vi "TemperatureTest.vi"() -> ()   [LabVIEW 2019]
uses:
  <vilib>/DAQmx/read.llb/DAQmx Read (Analog 1D DBL NChan 1Samp).vi
  <vilib>/DAQmx/create/channels.llb/DAQmx Create Channel (AI-Temperature-RTD).vi
  <vilib>/DAQmx/miscellaneous.llb/DAQmx Fill In Error Info.vi
panel:
  in  "rtd type":i32(ring)=10071 items=["Pt3750"=12481, "Pt3851"=10071, "Pt3911"=12482, "Pt3916"=10069, "Pt3920"=10053, "Pt3928"=12483, "Custom"=10137]
  in  "current excitation value":dbl=0.0009 format="%0.5f"
  in  "r0":dbl=100.0 format="%0.2f"
  in  "current excitation source":i32(ring)=10200 items=["Internal"=10200, "External"=10167, "None"=10230]
  in  "units":i32(ring)=10143 items=["Deg C"=10143, "Deg F"=10144, "Kelvins"=10325, "Deg R"=10145, "From Custom Scale"=10065]
  in  "physical channels":tag="PXI1Slot2/ai2"
  in  "resistance configuration":i32(ring)=2 items=["2-Wire"=2, "3-Wire"=3, "4-Wire"=4]
  in  "minimum value":dbl format="%0.2f"
  in  "maximum value":dbl=100.0 format="%0.2f"
  out "Thermometer":dbl(slide) scale=0.0..100.0
  out "Resultado":dbl
  in  "stop":bool
  out "Waveform Chart":dbl[](graph)
  # "Para el NI PXIe-4357"
  # "chanel 2 (ai2) for rtd"
  # "Pt3851 for rtd"
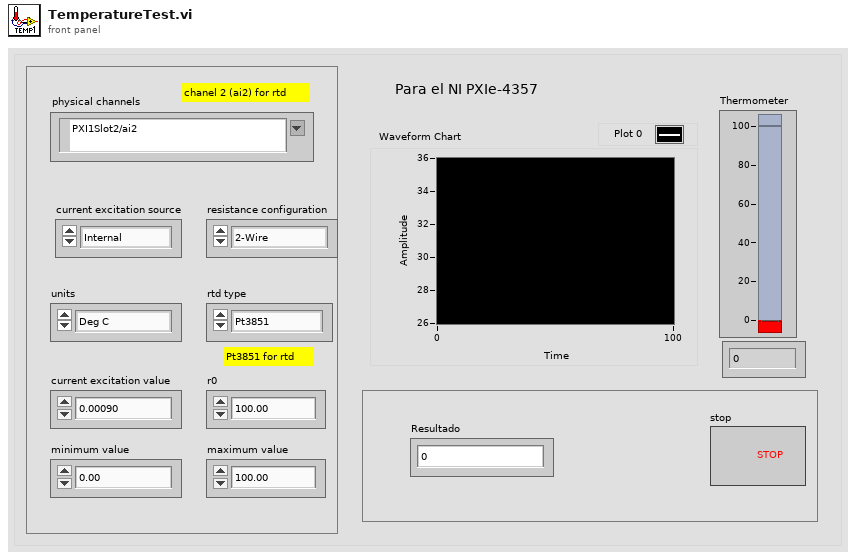
[diagram p1: front panel]
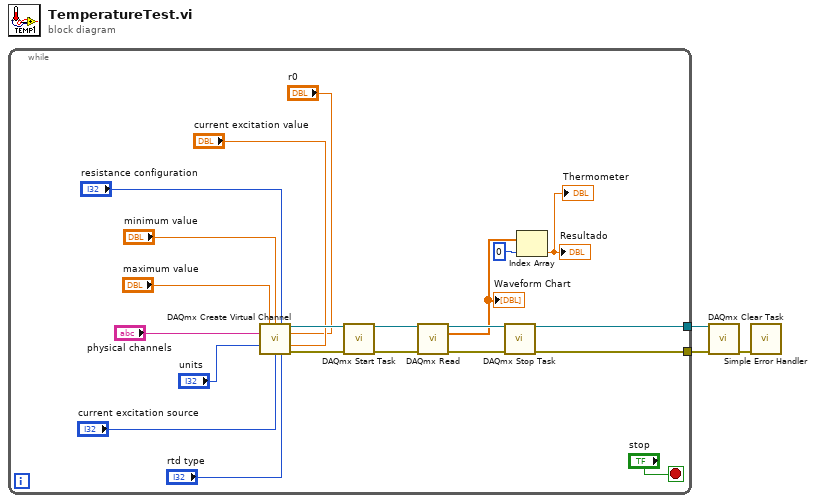
[diagram p0: block diagram]
diagram:
  n1 = while {
    tunnel: [w17] -> w2
    tunnel: [w16] -> w1
    stop <- "stop" stop-if-true
    n2 = call-poly <vilib>:"DAQmx Create Virtual Channel.vi"("maximum value"="maximum value", "minimum value"="minimum value", "resistance configuration"="resistance configuration", "physical channels"="physical channels", "r0"="r0", "units"="units", "current excitation value"="current excitation value", "current excitation source"="current excitation source", "rtd type"="rtd type") -> ("task out"=w24:refnum<k21>, "error out"=w23:errorcluster)  [unwired: 5 in]
    n3 = call <vilib>:"DAQmx Start Task.vi"("task/channels in"=w24, "error in"=w23) -> ("task out"=w22:refnum<k21>, "error out"=w21:errorcluster)  [unwired: 12 in]
    n4 = call-poly <vilib>:"DAQmx Read.vi"("task/channels in"=w22, "error in"=w21) -> ("task out"=w19:refnum<k21>, "data"=w15:dbl[], "error out"=w18:errorcluster)  [unwired: 11 in]
    "Waveform Chart" <- w15
    n5 = call <vilib>:"DAQmx Stop Task.vi"("task/channels in"=w19, "error in"=w18) -> ("task out"=w17:refnum<k21>, "error out"=w16:errorcluster)  [unwired: 12 in]
    n6 = Index Array(array=w15, index=0) -> (element=→"Resultado" →"Thermometer":dbl)
  }
  n7 = call <vilib>:"DAQmx Clear Task.vi"("task in"=w2, "error in"=w1) -> ("error out"=w3:errorcluster)  [unwired: 13 in]
  n8 = call <vilib>:"Simple Error Handler.vi"("error in (no error)"=w3) -> ()  [unwired: 4 in, 5 out]
